vi "getHeater.vi"(6 "Channel":i32, 8 "error in (no error)":errorcluster, 11 "Inst.TC in":refnum<class "Inst.TC.lvclass">) -> (0 "error out":errorcluster, 1 "Status":string, 2 "Current (mA)":dbl, 3 "Inst.TC out":refnum<class "Inst.TC.lvclass">)   [LabVIEW 2019, in "Inst.TC.lvclass"]
uses:
  Inst.TC.lvclass
  <userlib>/LevyLab/Instrument Framework/Instrument Types/Cryostat/Instrument.Cryostat.lvclass
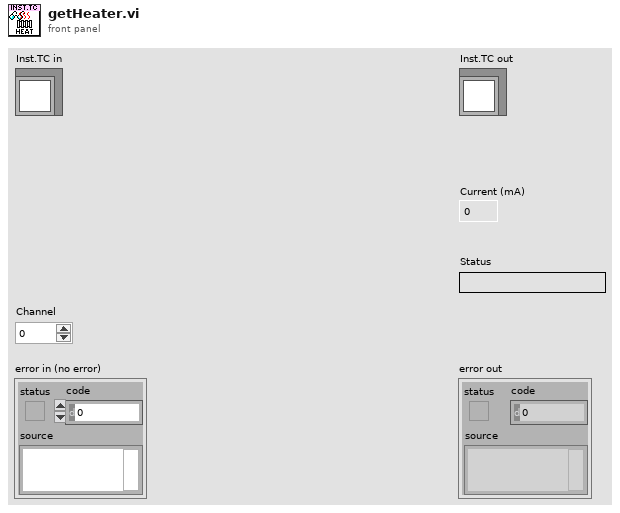
[diagram p1: front panel]
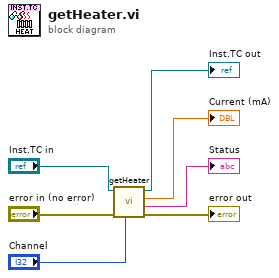
[diagram p0: block diagram]
diagram:
  n1 = call-parent "getHeater.vi"("Channel"="Channel", "error in (no error)"="error in (no error)", "Instrument.Cryostat in"="Inst.TC in") -> ("error out"=→"error out":errorcluster, "Status"=→"Status":string, "Current (A)"=→"Current (mA)":dbl, "Instrument.Cryostat out"=→"Inst.TC out":refnum<class "Inst.TC.lvclass">)  [unwired: 5 in]
